vi "Save_to_Matlab.vi"(6 "Path to PNG file":path, 7 "Line":string, 8 "Error in \n(no error)":errorcluster, 9 "Ball Touch":u32(colorbox), 10 "Band Touch":u32(colorbox), 11 "Balls coordinates":T1) -> (0 "Error out":errorcluster, 1 "Script of Analyse.m":string)   [LabVIEW 2019]
doc: "Save_to_Matlab.vi\nCreate the script of Analyse.m from Script.m (in current folder) and the coordinates of each balls.\nInput : -Path to PNG file\n -Band Touch containing the desired color for viewing the touched band in ScoreSheet.pdf\n -Ball Touch containing the desired color for viewing the touched ball in ScoreSheet.pdf\n -Line containing the desired linestyle for viewing the trajectory of balls in ScoreSheet.pdf\n -Balls coordinates in six differents vector\n -Error in\nOutput : -Script of Analyse.m in a string format\n -Error out"
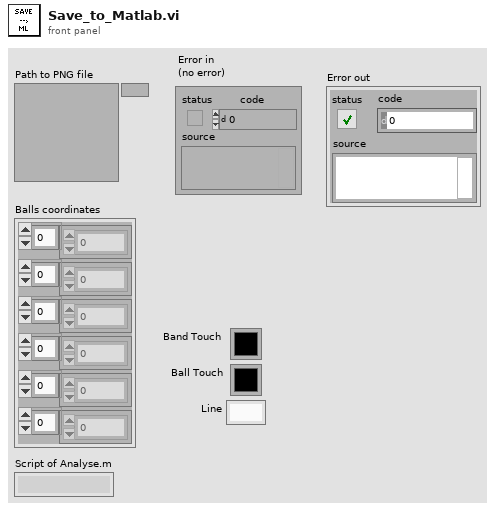
[diagram p1: front panel]
types:
  T1 = cluster{dbl[], dbl[], dbl[], dbl[], dbl[], dbl[]}
  T2 = typedef "imagedata.ctl" = cluster{"image type":i32, "image depth":i32, "image":u8[], "mask":u8[], "colors":u32[], "Rectangle":cluster{"left":i16, "top":i16, "right":i16, "bottom":i16}}
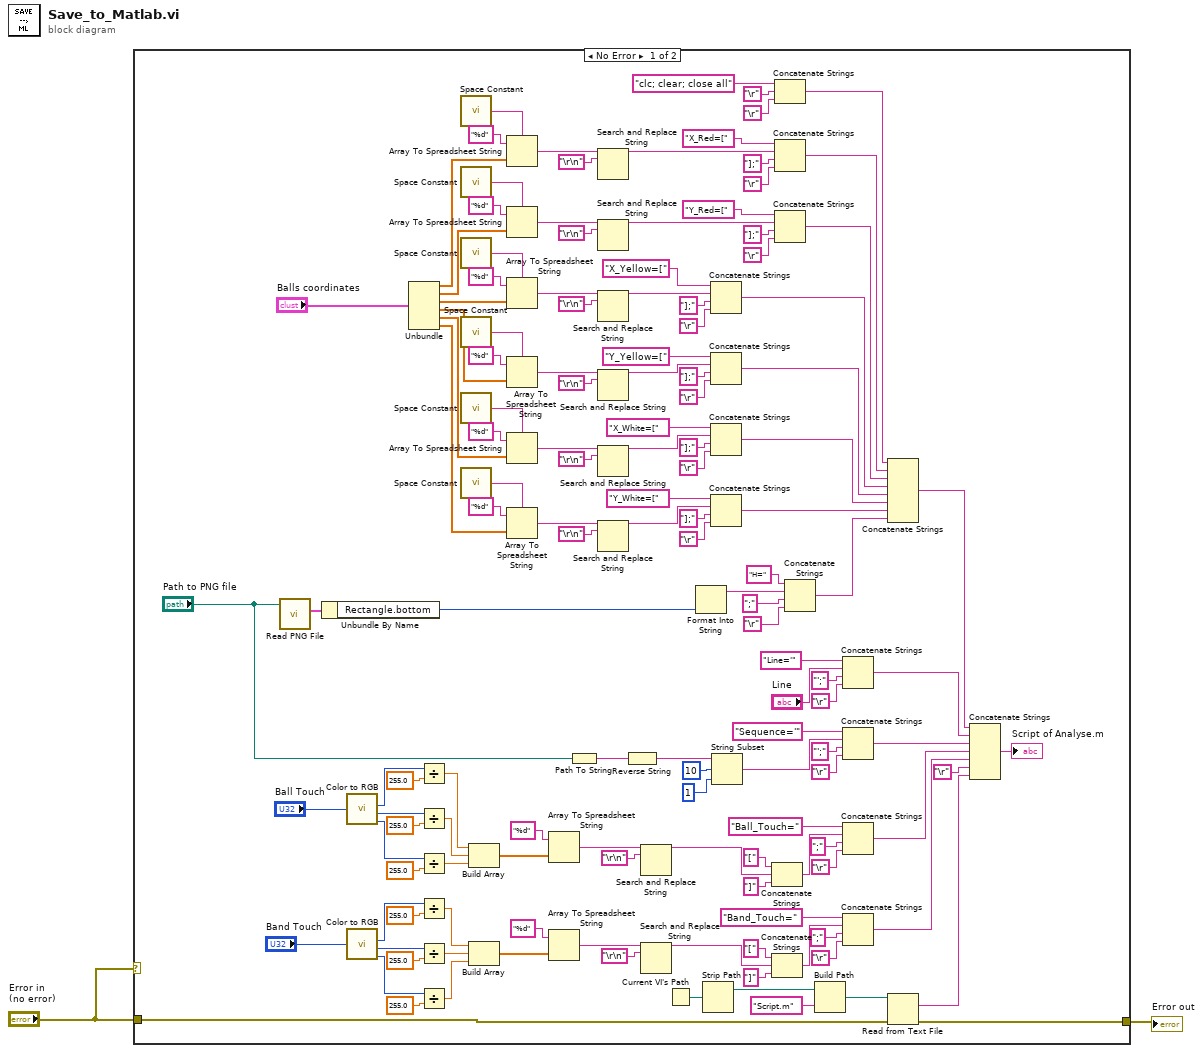
[diagram p0: block diagram]
diagram:
  n1 = case shown="No Error" "Error in \n(no error)" {
    tunnel: "Error in \n(no error)" -> [w5 w144]
    tunnel: [w4 w144] -> w2
    frame No Error {
      n2 = call <vilib>:"Read PNG File.vi"("path to PNG file"="Path to PNG file") -> ("image data"=w83:T2)  [unwired: 8 in, 2 out]
      n3 = Unbundle By Name(w83) -> ("Rectangle.bottom"=w82:i16)
      n4 = call <vilib>:"Color to RGB.vi"("Color"="Ball Touch") -> ("R"=w59:u8, "G"=w56:u8, "B"=w53:u8)  [unwired: 1 out]
      n5 = call <vilib>:"Color to RGB.vi"("Color"="Band Touch") -> ("R"=w50:u8, "G"=w47:u8, "B"=w44:u8)  [unwired: 1 out]
      n6 = Unbundle("Balls coordinates") -> (w137:dbl[], w136:dbl[], w135:dbl[], w134:dbl[], w133:dbl[], w132:dbl[])
      n7 = Divide(x=w59, y=255.0) -> (x/y=w58:dbl)
      n8 = Divide(x=w56, y=255.0) -> (x/y=w55:dbl)
      n9 = Divide(x=w53, y=255.0) -> (x/y=w52:dbl)
      n10 = Divide(x=w50, y=255.0) -> (x/y=w49:dbl)
      n11 = Divide(x=w47, y=255.0) -> (x/y=w46:dbl)
      n12 = Divide(x=w44, y=255.0) -> (x/y=w43:dbl)
      n13 = call <vilib>:"Space Constant.vi"() -> ("String"=w108:string)
      n14 = call <vilib>:"Space Constant.vi"() -> ("String"=w107:string)
      n15 = call <vilib>:"Space Constant.vi"() -> ("String"=w106:string)
      n16 = call <vilib>:"Space Constant.vi"() -> ("String"=w105:string)
      n17 = call <vilib>:"Space Constant.vi"() -> ("String"=w104:string)
      n18 = call <vilib>:"Space Constant.vi"() -> ("String"=w103:string)
      n19 = Build Array(w58, w55, w52) -> (w42:dbl[])
      n20 = Build Array(w49, w46, w43) -> (w41:dbl[])
      n21 = Array To Spreadsheet String(delimiter (Tab)=w108, array=w137, 3:"%d" ("format string")) -> (spreadsheet string=w100:string)
      n22 = Array To Spreadsheet String(delimiter (Tab)=w107, array=w136, 3:"%d" ("format string")) -> (spreadsheet string=w93:string)
      n23 = Array To Spreadsheet String(delimiter (Tab)=w106, array=w135, 3:"%d" ("format string")) -> (spreadsheet string=w91:string)
      n24 = Array To Spreadsheet String(delimiter (Tab)=w105, array=w134, 3:"%d" ("format string")) -> (spreadsheet string=w89:string)
      n25 = Array To Spreadsheet String(delimiter (Tab)=w104, array=w133, 3:"%d" ("format string")) -> (spreadsheet string=w87:string)
      n26 = Array To Spreadsheet String(delimiter (Tab)=w103, array=w132, 3:"%d" ("format string")) -> (spreadsheet string=w85:string)
      n27 = Array To Spreadsheet String(array=w42, 3:"%d" ("format string")) -> (spreadsheet string=w17:string)  [unwired: 1 in]
      n28 = Array To Spreadsheet String(array=w41, 3:"%d" ("format string")) -> (spreadsheet string=w14:string)  [unwired: 1 in]
      n29 = Path To String(path="Path to PNG file") -> (string=w62:string)
      n30 = Search and Replace String(input string=w100, search string="\r\n") -> (result string=w99:string)  [unwired: 6 in, 3 out]
      n31 = Search and Replace String(input string=w93, search string="\r\n") -> (result string=w92:string)  [unwired: 6 in, 3 out]
      n32 = Search and Replace String(input string=w91, search string="\r\n") -> (result string=w90:string)  [unwired: 6 in, 3 out]
      n33 = Search and Replace String(input string=w89, search string="\r\n") -> (result string=w88:string)  [unwired: 6 in, 3 out]
      n34 = Search and Replace String(input string=w87, search string="\r\n") -> (result string=w86:string)  [unwired: 6 in, 3 out]
      n35 = Search and Replace String(input string=w85, search string="\r\n") -> (result string=w84:string)  [unwired: 6 in, 3 out]
      n36 = Reverse String(1:w62) -> (0:w61:string)
      n37 = Search and Replace String(input string=w17, search string="\r\n") -> (result string=w16:string)  [unwired: 6 in, 3 out]
      n38 = Search and Replace String(input string=w14, search string="\r\n") -> (result string=w13:string)  [unwired: 6 in, 3 out]
      n39 = Current VI's Path() -> (path=w11:path)
      n40 = Format Into String(w82) -> (resulting string=w80:string)  [unwired: 3 in, 1 out]
      n41 = Strip Path(path=w11) -> (stripped path=w10:path)  [unwired: 1 out]
      n42 = Concatenate Strings("X_Yellow=[" ("string"), w90, "];" ("string"), "\r") -> (w117:string)
      n43 = Concatenate Strings("Y_Yellow=[" ("string"), w88, "];" ("string"), "\r") -> (w116:string)
      n44 = Concatenate Strings("X_White=[" ("string"), w86, "];" ("string"), "\r") -> (w115:string)
      n45 = Concatenate Strings("Y_White=[" ("string"), w84, "];" ("string"), "\r") -> (w114:string)
      n46 = String Subset(string=w61, offset (0)=10, length (rest)=1 ("length (rest)")) -> (substring=w35:string)
      n47 = Concatenate Strings("[" ("string"), w16, "]" ("string")) -> (w28:string)
      n48 = Concatenate Strings("[" ("string"), w13, "]" ("string")) -> (w27:string)
      n49 = Concatenate Strings("clc; clear; close all" ("string"), "\r", "\r") -> (w73:string)
      n50 = Concatenate Strings("X_Red=[" ("string"), w99, "];" ("string"), "\r") -> (w119:string)
      n51 = Concatenate Strings("Y_Red=[" ("string"), w92, "];" ("string"), "\r") -> (w118:string)
      n52 = Concatenate Strings("H=" ("string"), w80, ";" ("string"), "\r") -> (w77:string)
      n53 = Build Path(base path=w10, name or relative path="Script.m") -> (appended path=w9:path)
      n54 = Concatenate Strings("Line='" ("string"), "Line", "';" ("string"), "\r") -> (w24:string)
      n55 = Concatenate Strings("Sequence='" ("string"), w35, "';" ("string"), "\r") -> (w23:string)
      n56 = Concatenate Strings("Ball_Touch=" ("string"), w28, ";" ("string"), "\r") -> (w22:string)
      n57 = Concatenate Strings("Band_Touch=" ("string"), w27, ";" ("string"), "\r") -> (w21:string)
      n58 = Concatenate Strings(w73, w119, w118, w117, w116, w115, w114, w77) -> (w65:string)
      n59 = Read from Text File(file (use dialog)=w9, error in=w5) -> (text=w8:string, error out=w4:errorcluster)  [unwired: 2 in, 2 out]
      n60 = Concatenate Strings(w65, w24, w23, w22, w21, "\r", w8) -> (→"Script of Analyse.m":string)
    }
    frame Error {
    }
  }
  "Error out" <- w2
